vi "NML Bus Scan Oxford IPS.vi"(3 "error out":errorcluster, 4 "String Read 2":string, 5 "VISA session":refnum<visa-resource-name>) -> (0 "error IO":errorcluster, 1 "String Read":string, 2 "VISA Resource Name":refnum<visa-resource-name>)   [LabVIEW 2019]
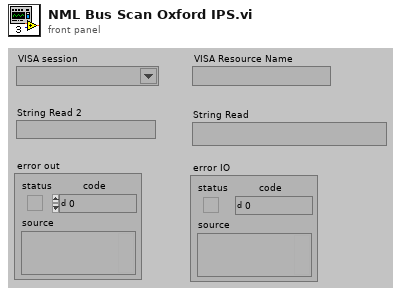
[diagram p1: front panel]
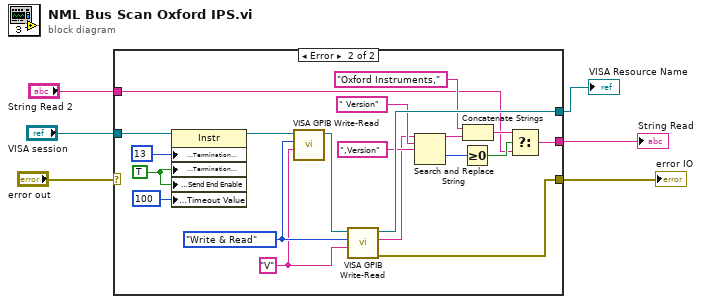
[diagram p0: block diagram]
diagram:
  n1 = case shown="Error" "error out" {
    selector: "error out" -> [w7 _]
    tunnel: "VISA session" -> [w9 w26]
    tunnel: [w9 w28] -> w3
    tunnel: [w8 w13] -> w5
    tunnel: "String Read 2" -> [w8 w10]
    tunnel: [w7 w29] -> w6
    frame No Error {
    }
    frame Error {
      w25 = enum16{"Write", "Read", "Write & Read"}."Write & Read" ("Action")
      w21 = TRUE ("Message Based Settings:Termination Character Enable")
      w22 = "V" ("String to Write")
      n2 = property class="Instr"(reference=w26, "Message Based Settings:Termination Character"=u8 13, "Message Based Settings:Termination Character Enable"=w21, "Message Based Settings:Send End Enable"=w21, "General Settings:Timeout Value"=u32 100) -> (reference out=w24:refnum<visa-resource-name>)  [unwired: 1 in, 1 out]
      n3 = call "VISA GPIB Write-Read.vi"("Command"=w22, "Action"=w25, "VISA resource name"=w24) -> ("dup VISA Session"=w23:refnum<visa-resource-name>)  [unwired: 5 in, 3 out]
      n4 = call "VISA GPIB Write-Read.vi"("Command"=w22, "Action"=w25, "VISA resource name"=w23) -> ("error out"=w29:errorcluster, "String Returned"=w17:string, "dup VISA Session"=w28:refnum<visa-resource-name>)  [unwired: 5 in, 1 out]
      n5 = Search and Replace String(input string=w17, search string=" Version", replace string=",Version" ("replace string (\"\")")) -> (result string=w15:string, offset past replacement=w14:i32)  [unwired: 5 in, 2 out]
      n6 = Greater Or Equal To 0?(x=w14) -> (x >= 0?=w11:bool)
      n7 = Concatenate Strings("Oxford Instruments," ("string"), w15) -> (w12:string)
      n8 = Select(t=w12, s=w11, f=w10) -> (s? t:f=w13:string)
    }
  }
  "error IO" <- w6
  "String Read" <- w5
  "VISA Resource Name" <- w3
